vi "Read.vi"(8 "Error In":errorcluster, 11 "SerialComm in":refnum<class "SerialComm.lvclass">) -> (0 "Error Out":errorcluster, 3 "SerialComm out":refnum<class "SerialComm.lvclass">)   [LabVIEW 2016, in "SerialComm.lvclass"]
uses:
  SerialComm.lvclass
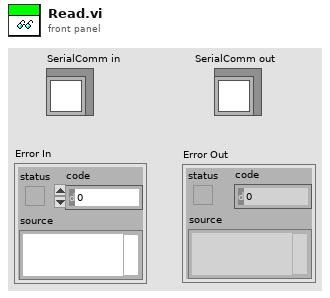
[diagram p1: front panel]
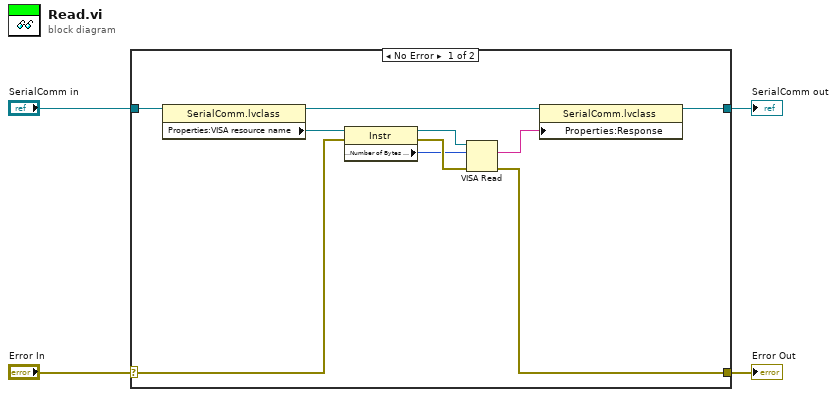
[diagram p0: block diagram]
diagram:
  n1 = case shown="No Error" "Error In" {
    selector: "Error In" -> [w11 w16]
    tunnel: [w8 w16] -> w3
    tunnel: [w7 w15] -> w1
    tunnel: "SerialComm in" -> [w14 w15]
    frame No Error {
      n2 = property class="SerialComm.lvclass"(reference=w14) -> (reference out=w13:refnum<class "SerialComm.lvclass">, "Properties:VISA resource name"=w12:refnum<visa-resource-name>)  [unwired: 1 in, 1 out]
      n3 = property class="Instr"(reference=w12, error in=w11) -> (reference out=w10:refnum<visa-resource-name>, error out=w9:errorcluster, "Serial Settings:Number of Bytes at Serial Port"=w5:u32)
      n4 = VISA Read(VISA resource name=w10, byte count=w5, error in (no error)=w9) -> (read buffer=w6:string, error out=w8:errorcluster)  [unwired: 2 out]
      n5 = property class="SerialComm.lvclass"(reference=w13, "Properties:Response"=w6) -> (reference out=w7:refnum<class "SerialComm.lvclass">)  [unwired: 1 in, 1 out]
    }
    frame Error {
    }
  }
  "Error Out" <- w3
  "SerialComm out" <- w1
